vi "ge_GraphTblFGV.vi"(3 "ge_DAQManDefinitions":T1, 4 "Cal Ref":cluster{"EU RMS":dbl, "dB":bool}, 5 "ItemNames":string[][](array[string]), 6 "RMS Value":dbl, 7 "GrphTblCmnds":T4, 8 "error in":errorcluster, 9 "Legend LB":i32[](array[numeric]), 10 "Wfm In":waveform(dbl)[](array[waveform]), 11 "Init Info":T2) -> (0 "error out":errorcluster, 1 "Cell Contents":T3(array[cluster]), 2 "Wfm Out":waveform(dbl)[](array[waveform]))   [LabVIEW 2018]
uses:
  ge_GrphTblCmnds.ctl
  Classes/Measurements/Class Dynamic/Dynamic.lvclass
  C:/Users/Jeff Tipps/Documents/DAQMan/source/Classes/Measurements/Class Channel/Channel.lvclass
  Common/Controls/DAQMan Definitions.ctl
  Custom Ctrls/ge_FPCtrlRefLabel.ctl
  <vilib>/Utility/miscctls.llb/LVRowAndColumnTypeDef.ctl
  <vilib>/addons/_NISVFA/_Shared subVIs/Controls/svc_Channel Info.ctl
  <vilib>/addons/_NISVFA/_Shared subVIs/Controls/svc_Engineering Units Text Ring.ctl
  <vilib>/addons/_NISVFA/_Shared subVIs/Controls/svc_Weighting Filter Text Ring.ctl
  Custom Ctrls/ge_MeasType.ctl
  Common/Controls/HeaderNames.ctl
  <vilib>/addons/Sound and Vibration/svt_Calibration/SVL Scale Voltage to EU (1 Ch).vi
  <vilib>/addons/_NISVFA/_Shared subVIs/Common/svc_Set SV Channel Info.vi
  <vilib>/addons/_NISVFA/_Shared subVIs/Common/svc_Set SV Channel Info (variant).vi
  <vilib>/addons/_NISVFA/_Shared subVIs/Common/SVL Set dB Reference (variant).vi
  Classes/Measurements/Class Channel/Read Unit_EU.vi
  Classes/Measurements/Class Dynamic/Read dB Ref.vi
  <vilib>/addons/_NISVFA/_Shared subVIs/Common/svc_Engineering Units to Unit Label.vi
  <vilib>/addons/_NISVFA/_Shared subVIs/Common/svc_Compute Scale Factor to Convert V to EU.vi
  <vilib>/addons/_NISVFA/_Shared subVIs/Common/svc_Compute Scale Factor to Convert C to EU.vi
  <vilib>/addons/_NISVFA/_Shared subVIs/Common/svc_Set dB ref if Pascal.vi
  <vilib>/addons/_NISVFA/_Shared subVIs/Common/svc_Caller VI Returned in Error Source.vi
  Classes/Measurements/Class Dynamic/Read Cal Mag.vi
  Classes/Measurements/Class Dynamic/Read Cal Units.vi
  <vilib>/addons/Sound and Vibration/svt_Calibration/SoundVib_Calibration.lvlib
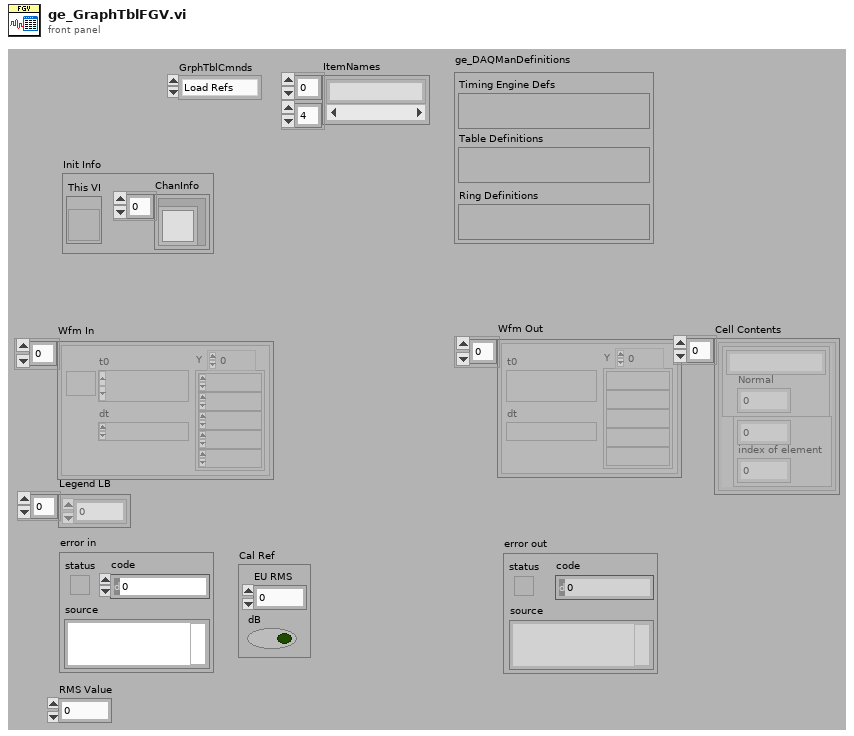
[diagram p1: front panel]
types:
  T1 = typedef "DAQMan Definitions.ctl" = cluster{"Timing Engine Defs":variant, "Table Definitions":variant, "Ring Definitions":variant}
  T2 = cluster{"This VI":refnum<vi>, "ChanInfo":refnum<class "Dynamic.lvclass">[]}
  T3 = cluster{cluster{string, "Normal":u32}, cluster{i32, "index of element":i32}}[]
  T4 = typedef "ge_GrphTblCmnds.ctl" = enum16{"Load Refs", "Init FP", "Active Plot", "CalRef", "AcceptCal", "Scale Wfm", "Update RMS", "Update Sens", "Get Sens", "Shutdown"}
  T5 = typedef "LVRowAndColumnTypeDef.ctl" = cluster{"Row":i32, "Column":i32}
  T6 = typedef "svc_Channel Info.ctl" = cluster{"sensor sensitivity":dbl, "engineering units":T7, "dB reference":dbl, "custom label":string, "weighting filter":T8, "pregain":dbl}
  T7 = typedef "svc_Engineering Units Text Ring.ctl" = u16
  T8 = typedef "svc_Weighting Filter Text Ring.ctl" = u16
  T9 = typedef "HeaderNames.ctl" = enum16{"Channel", "Device", "Spacer", "Description", "MB", "Range", "Terminal", "Coupling", "Thresh (V)", "Pulse/Rev", "Slope", "Min EU", "Min RPM", "mV/EU", "Iex", "Temp Units", "Type", "CJC Src", "CJC Val", "Ro", "Wire Cfg", "Strain Mode", "Vex", "Bridge Type", "GF", "Gauge Res", "Poisson", "Lead Res", "Init Strain", "GAF", "Scale", "Offset", "Unit (EU)", "dB?", "dB Ref", "Cal Mag", "Cal Units", "Max Temp", "Min Temp", "Max Strain", "Min Strain"}
  T10 = typedef "ge_MeasType.ctl" = enum16{"Voltage", "Frequency", "Tachometer", "Dynamic", "Thermocouple", "RTD", "Strain", "Current", "Resistance"}
  T11 = typedef "ge_FPCtrlRefLabel.ctl" = cluster{"Label Array":string[], "Ref Array":refnum<vi>[]}
  T12 = cluster{cluster{string, "Coerced":u32}, cluster{i32, "index of element":i32}}
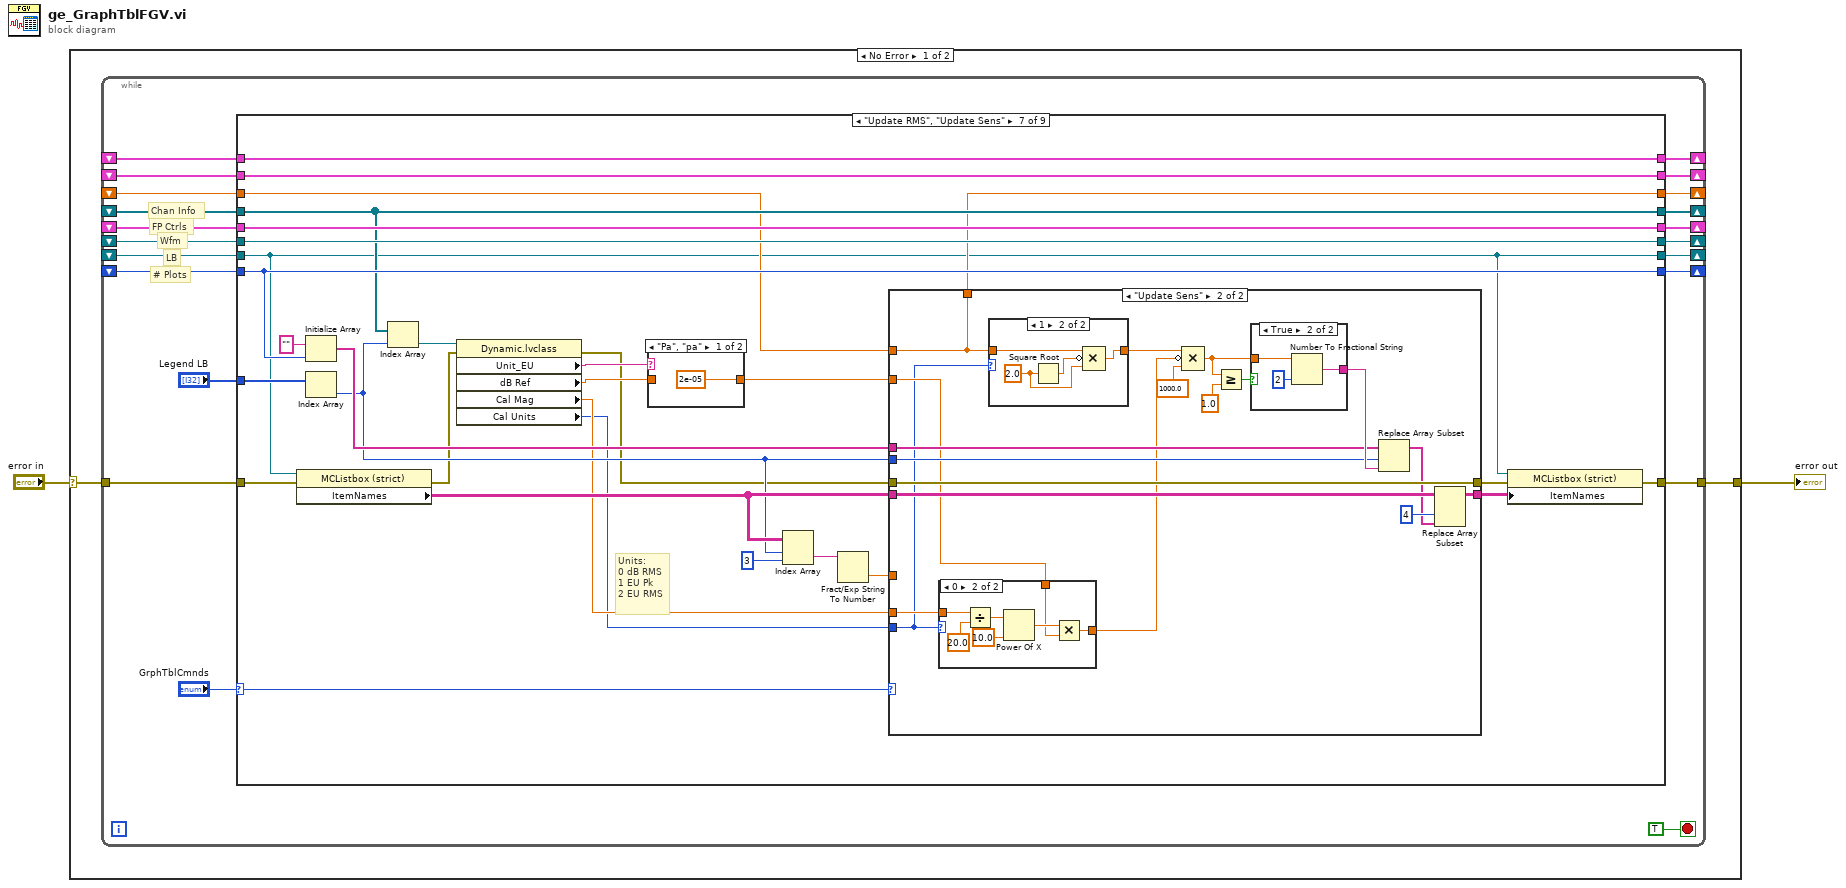
[diagram p0: block diagram]
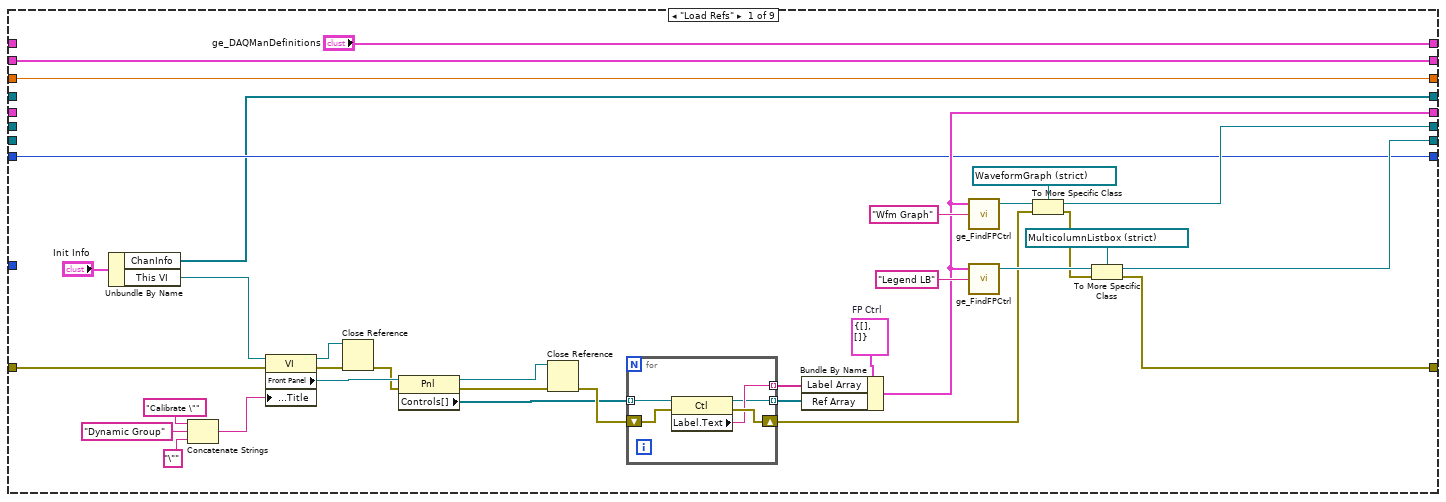
[diagram p2: hidden frame]
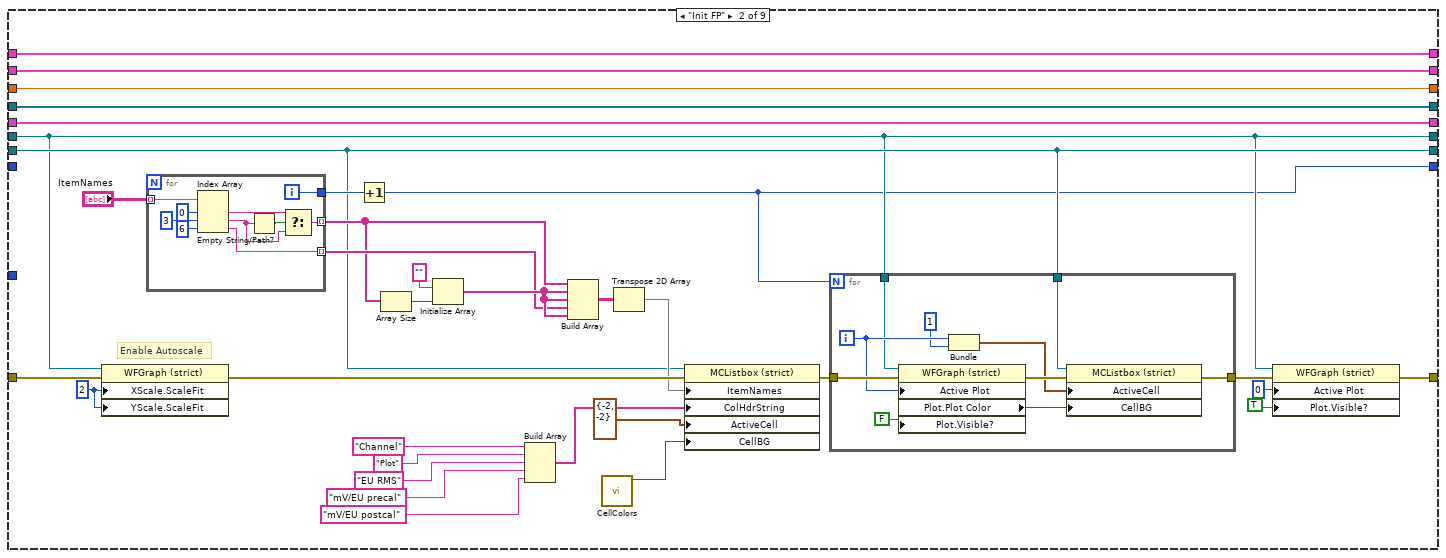
[diagram p3: hidden frame]
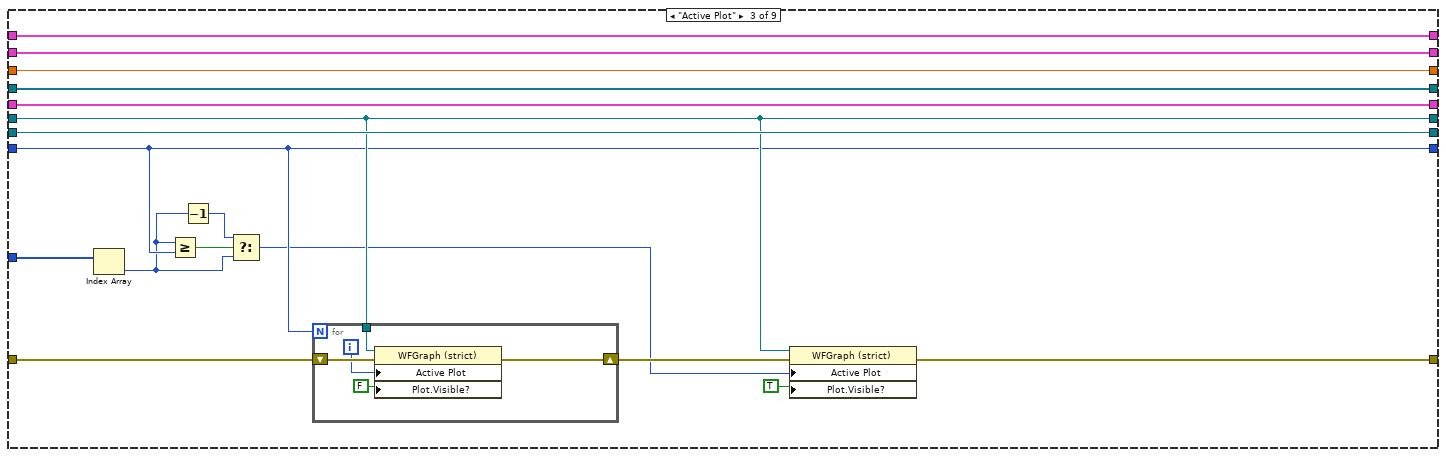
[diagram p4: hidden frame]
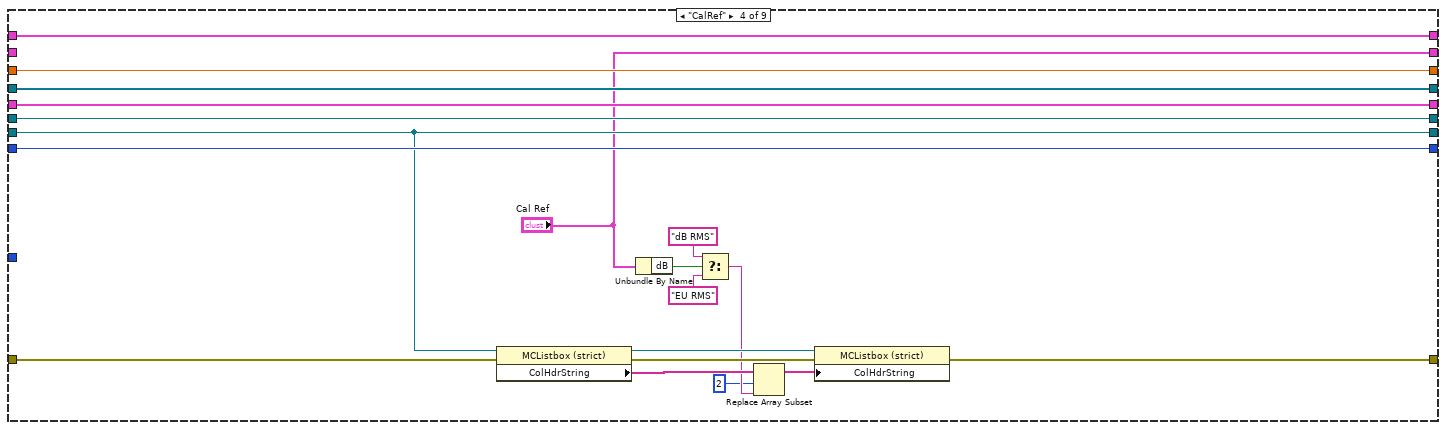
[diagram p5: hidden frame]
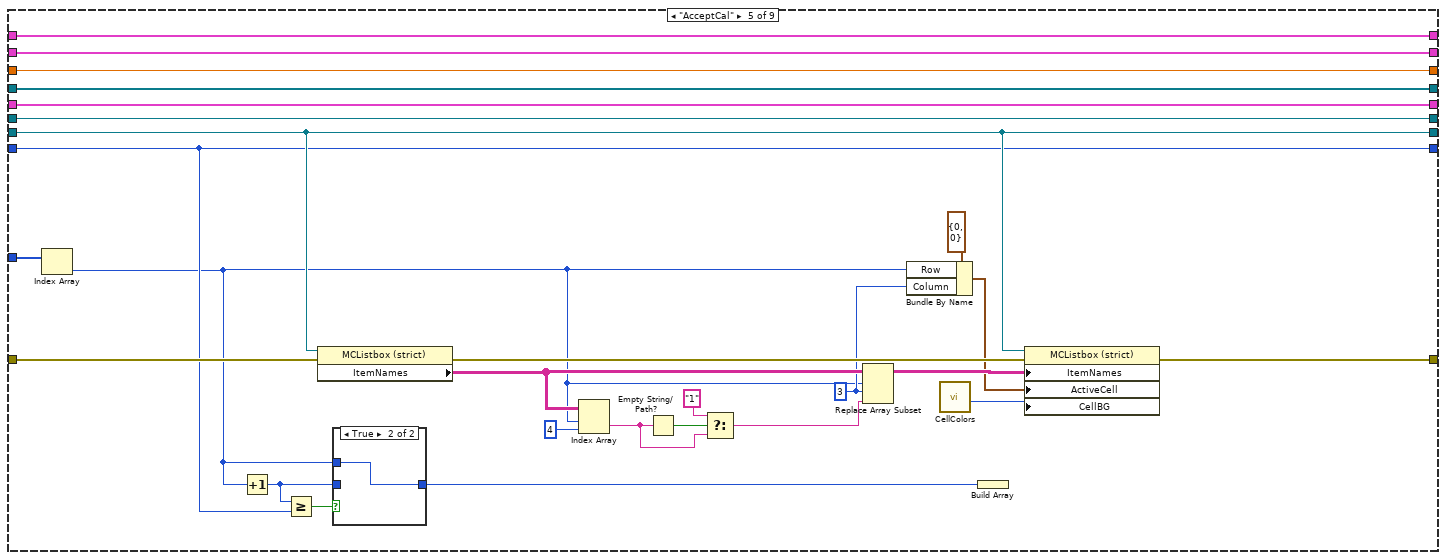
[diagram p6: hidden frame]
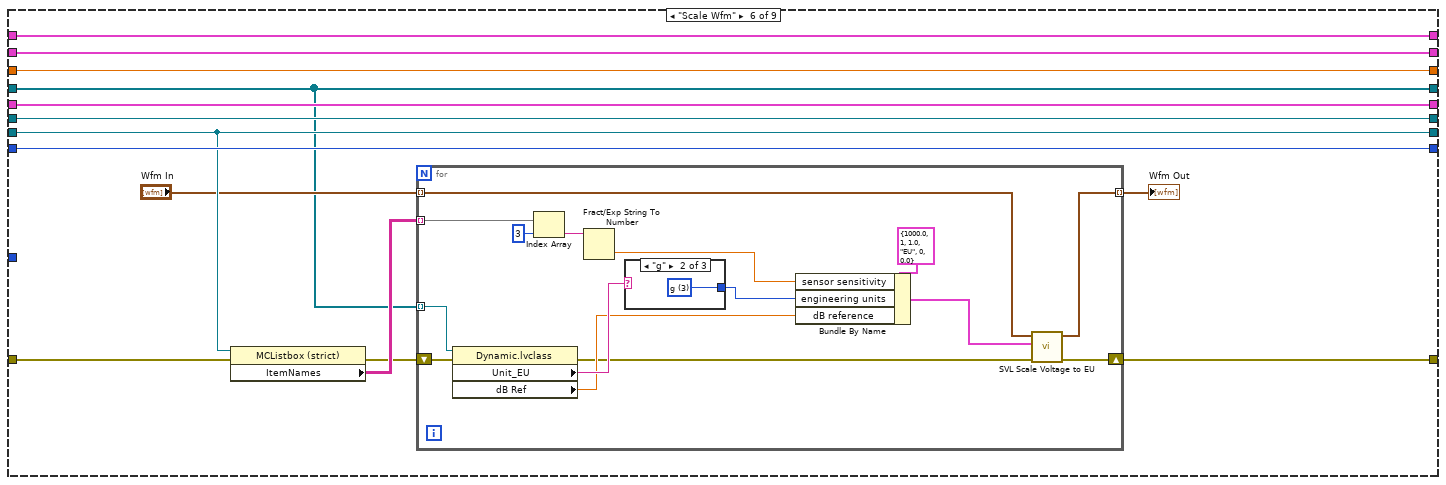
[diagram p8: hidden frame]
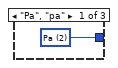
[diagram p9: hidden frame]
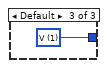
[diagram p10: hidden frame]
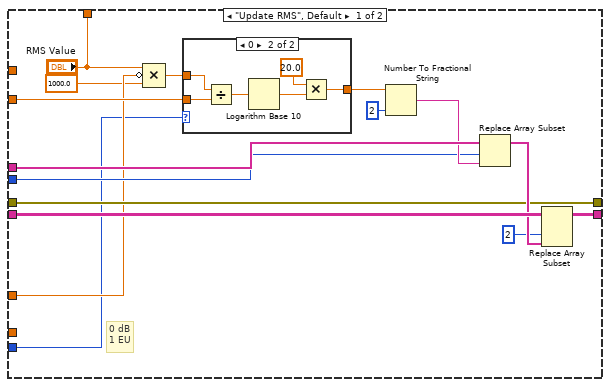
[diagram p11: hidden frame]
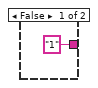
[diagram p15: hidden frame]
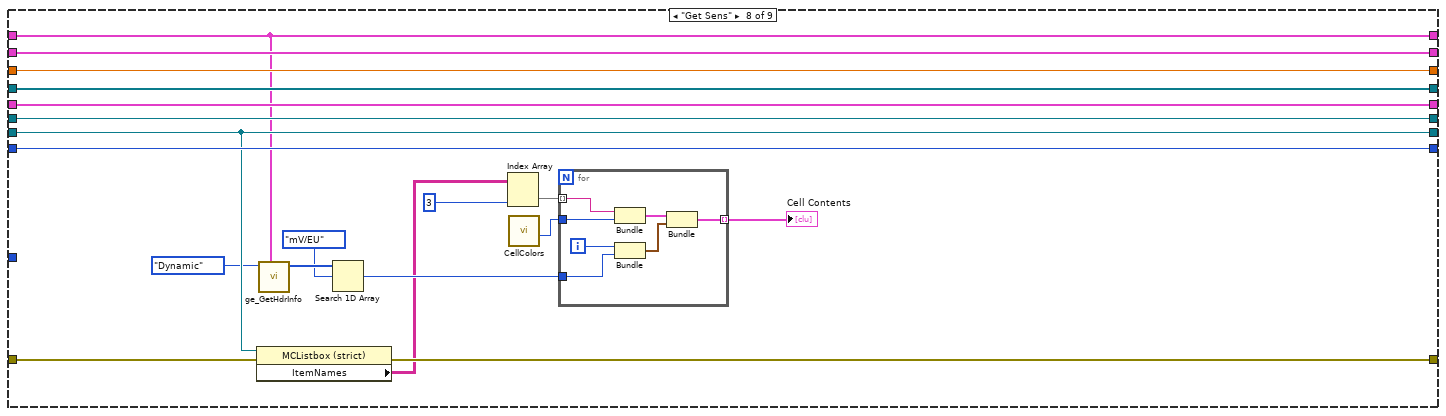
[diagram p17: hidden frame]
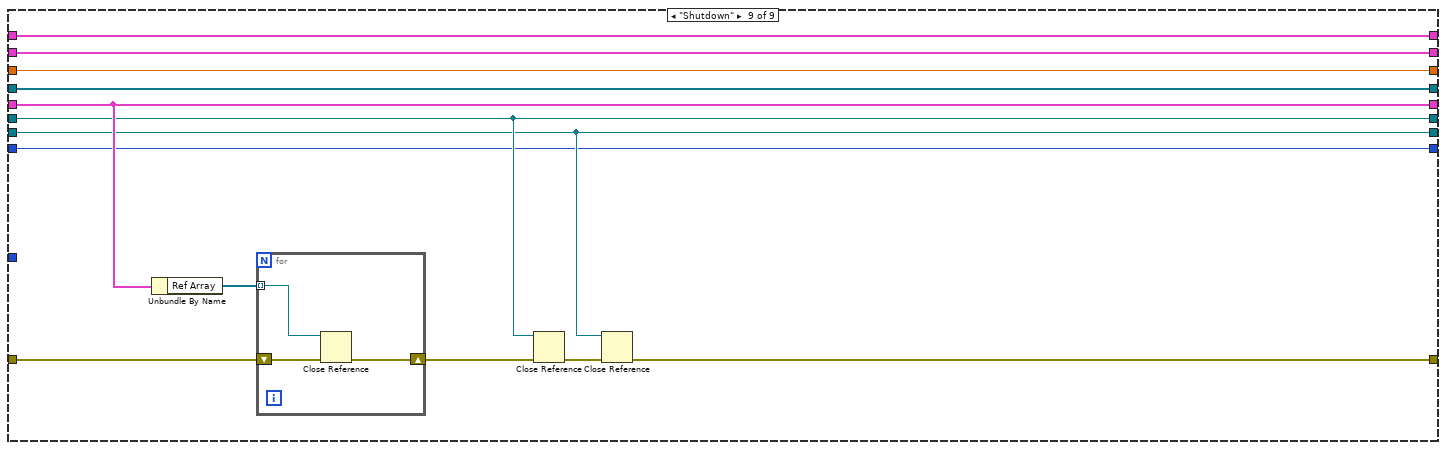
[diagram p18: hidden frame]
diagram:
  n1 = case shown="No Error" "error in" {
    selector: "error in" -> [w4 w353]
    tunnel: [w3 w353] -> w1
    frame No Error {
      n2 = while {
        tunnel: w4 -> [w25]
        tunnel: [w22] -> w3
        shift-right: [w21] -> _
        shift-left: _ -> [w19]
        shift-right: [w20] -> _
        shift-left: _ -> [w18]
        shift-right: [w17] -> _
        shift-left: _ -> [w16]
        shift-right: [w15] -> _
        shift-left: _ -> [w14]
        shift-right: [w12] -> _
        shift-left: _ -> [w11]
        shift-right: [w10] -> _
        shift-left: _ -> [w9]
        shift-right: [w8] -> _
        shift-left: _ -> [w7]
        shift-right: [w6] -> _
        shift-left: _ -> [w5]
        stop <- TRUE stop-if-true
        # "FP Ctrls"
        # "Chan Info"
        # "# Plots"
        # "Wfm"
        # "LB"
        n3 = case shown="\"Update RMS\", \"Update Sens\"" "GrphTblCmnds" {
          selector: "GrphTblCmnds" -> [_ _ _ _ _ _ w237 _ _]
          tunnel: w25 -> [w48 w97 w132 w154 w180 w199 w225 w324 w349]
          tunnel: [w38 w71 w135 w150 w179 w191 w243 w323 w344] -> w22
          tunnel: [w37 w72 w130 w158 w175 w201 w249 w328 w343] -> w21
          tunnel: [w35 w76 w133 w153 w178 w198 w236 w322 w342] -> w20
          tunnel: w19 -> [_ w72 w130 w158 w175 w201 w249 w328 w343]
          tunnel: w18 -> [_ w76 w133 w153 w178 w198 w236 w322 w342]
          tunnel: [w34 w98 w134 w159 w186 w202 w250 w329 w347] -> w17
          tunnel: w16 -> [_ w98 w134 w159 w186 w202 w250 w329 w347]
          tunnel: [w33 w70 w126 w157 w170 w200 w247 w327 w341] -> w15
          tunnel: w14 -> [w33 _ w126 w157 w170 w200 w247 w327 w341]
          tunnel: "Legend LB" -> [_ _ w127 _ w181 _ w246 _ _]
          tunnel: [w29 w69 w129 w156 w177 w190 w242 w326 w340] -> w12
          tunnel: w11 -> [_ w69 w129 w156 w177 w190 w242 w326 w340]
          tunnel: [w32 w68 w128 w155 w176 w195 w240 w325 w339] -> w10
          tunnel: w9 -> [w32 w68 w128 w155 w176 w195 w238 w325 w339]
          tunnel: [w28 w67 w120 "Cal Ref" w161 w194 w230 w316 w338] -> w8
          tunnel: w7 -> [w28 w67 w120 _ w161 w194 w230 w316 w338]
          tunnel: ["ge_DAQManDefinitions" w66 w119 w141 w160 w189 w229 w314 w337] -> w6
          tunnel: w5 -> [_ w66 w119 w141 w160 w189 w229 w314 w337]
          frame "Load Refs" {
            w49 = T11 {"Label Array"=[], "Ref Array"=[]}  # FP Ctrl
            n4 = Unbundle By Name("Init Info") -> ("ChanInfo"=w29:refnum<class "Dynamic.lvclass">[], "This VI"=w30:refnum<vi>)
            n5 = Concatenate Strings("Calibrate \"", "Dynamic Group" ("string"), "\"") -> (w52:string)
            n6 = property class="VI"(reference=w30, error in=w48, "Front Panel.Title"=w52) -> (reference out=w46:refnum<vi>, error out=w47:errorcluster, "Front Panel"=w56:refnum<vi>)
            n7 = Close Reference(reference=w46, error in (no error)=w47) -> (error out=w45:errorcluster)
            n8 = property class="Pnl"(reference=w56, error in=w45) -> (reference out=w60:refnum<vi>, error out=w58:errorcluster, "Controls[]"=w57:refnum<vi>[])
            n9 = Close Reference(reference=w60, error in (no error)=w58) -> (error out=w59:errorcluster)
            n10 = for {
              tunnel: w57 -> [w65] mode=indexing
              shift-right: [w63] -> w40
              shift-left: w59 -> [w64]
              tunnel: [w62] -> w51 mode=indexing
              tunnel: [w61] -> w50 mode=indexing
              n11 = property class="Ctl"(reference=w65, error in=w64) -> (reference out=w61:refnum<vi>, error out=w63:errorcluster, "Label.Text"=w62:string)
            }
            n12 = Bundle By Name(cluster=w49, "Label Array"=w51, "Ref Array"=w50) -> (w34:T11)
            n13 = call "ge_FindFPCtrl.vi"("Ctrl Name"="Wfm Graph", "FP Ctrl"=w34) -> ("Ctrl Ref"=w42:refnum<vi>)  [unwired: 3 in]
            n14 = call "ge_FindFPCtrl.vi"("Ctrl Name"="Legend LB", "FP Ctrl"=w34) -> ("Ctrl Ref"=w41:refnum<vi>)  [unwired: 3 in]
            n15 = To More Specific Class(target class=refnum<vi> refnum ("Wfm Graph"), reference=w42, error in=w40) -> (specific class reference=w37:refnum<vi>, error out=w39:errorcluster)
            n16 = To More Specific Class(target class=refnum<vi> refnum ("Legend LB"), reference=w41, error in=w39) -> (specific class reference=w35:refnum<vi>, error out=w38:errorcluster)
          }
          frame "Init FP" {
            w96 = u8 2 ("X Scale.Scale Fit")
            # "Enable Autoscale"
            n17 = property on="Property Node" class="WFGraph (strict)"(reference=w72, error in=w97, "XScale.ScaleFit"=w96, "YScale.ScaleFit"=w96) -> (error out=w95:errorcluster)  [unwired: 1 out]
            n18 = for {
              tunnel: "ItemNames" -> [w116] mode=indexing
              tunnel: [w117] -> w83 mode=indexing
              tunnel: [w110] -> w85 mode=indexing
              tunnel: [w109] -> w79
              i -> [w109]
              n19 = Index Array(array=w116, index #1=0 ("index"), index #2=3 ("index"), index #3=6 ("index")) -> (element #1=w114:string, element #2=w113:string, element #3=w110:string)
              n20 = Empty String/Path?(string/path=w113) -> (empty?=w118:bool)
              n21 = Select(t=w114, s=w118, f=w113) -> (s? t:f=w117:string)
            }
            n22 = Increment(x=w79) -> (x+1=w70:i32)
            n23 = Array Size(array=w83) -> (size(s)=w82:i32)
            n24 = Initialize Array("", w82) -> (w86:string[])
            n25 = Build Array("Channel", "Plot", "EU RMS", "mV/EU precal" ("element"), "mV/EU postcal" ("element")) -> (w89:string[])
            n26 = Build Array(w83, w86, w86, w85, w86) -> (w84:string[][])
            n27 = call "CellColors.vi"() -> ("Normal"=w87:u32)  [unwired: 8 in, 3 out]
            n28 = Transpose 2D Array(2D array=w84) -> (transposed array=w77:string[][])
            n29 = property on="Property Node" class="MCListbox (strict)"(reference=w76, error in=w95, "ItemNames"=w77, "ColHdrString"=w89, "ActiveCell"=T5 {"Row"=-2, "Column"=-2} ("Active Cell:Active Cell"), "CellBG"=w87) -> (error out=w78:errorcluster)  [unwired: 1 out]
            n30 = for {
              N: w70 -> [_]
              tunnel: [w108] -> w73
              tunnel: w78 -> [w106]
              tunnel: w72 -> [w100]
              tunnel: w76 -> [w99]
              i -> [w104]
              n31 = property on="Property Node" class="WFGraph (strict)"(reference=w100, error in=w106, "Active Plot"=w104, "Plot.Visible?"=FALSE ("Plot.Visible")) -> (error out=w107:errorcluster, "Plot.Plot Color"=w105:u32)  [unwired: 1 out]
              n32 = Bundle(w104, 1) -> (w102:cluster{i32, i32})  [unwired: 1 in]
              n33 = property on="Property Node" class="MCListbox (strict)"(reference=w99, error in=w107, "ActiveCell"=w102, "CellBG"=w105) -> (error out=w108:errorcluster)  [unwired: 1 out]
            }
            n34 = property on="Property Node" class="WFGraph (strict)"(reference=w72, error in=w73, "Active Plot"=u32 0, "Plot.Visible?"=TRUE ("Plot.Visible")) -> (error out=w71:errorcluster)  [unwired: 1 out]
          }
          frame "Active Plot" {
            n35 = Index Array(array=w127) -> (element=w124:i32)  [unwired: 1 in]
            n36 = Greater Or Equal?(x=w124, y=w126) -> (x >= y?=w125:bool)
            n37 = Decrement(x=w124) -> (x-1=w123:i32)
            n38 = Select(t=w123, s=w125, f=w124) -> (s? t:f=w122:i32)
            n39 = for {
              N: w126 -> [_]
              shift-right: [w139] -> w131
              shift-left: w132 -> [w140]
              tunnel: w130 -> [w136]
              i -> [w137]
              n40 = property on="Property Node" class="WFGraph (strict)"(reference=w136, error in=w140, "Active Plot"=w137, "Plot.Visible?"=FALSE ("Plot.Visible")) -> (error out=w139:errorcluster)  [unwired: 1 out]
            }
            n41 = property on="Property Node" class="WFGraph (strict)"(reference=w130, error in=w131, "Active Plot"=w122, "Plot.Visible?"=TRUE ("Plot.Visible")) -> (error out=w135:errorcluster)  [unwired: 1 out]
          }
          frame "CalRef" {
            n42 = property on="Property Node" class="MCListbox (strict)"(reference=w153, error in=w154) -> (reference out=w147:refnum<vi>, error out=w151:errorcluster, "ColHdrString"=w148:string[])
            n43 = Unbundle By Name("Cal Ref") -> ("dB"=w149:bool)
            n44 = Select(t="dB RMS", s=w149, f="EU RMS") -> (s? t:f=w146:string)
            n45 = Replace Array Subset(array=w148, new element=w146, index=2) -> (w142:string[])
            n46 = property on="Property Node" class="MCListbox (strict)"(reference=w147, error in=w151, "ColHdrString"=w142) -> (error out=w150:errorcluster)  [unwired: 1 out]
          }
          frame "AcceptCal" {
            w173 = 3 ("disabled index (col)")
            n47 = Index Array(array=w181) -> (element=w168:i32)  [unwired: 1 in]
            n48 = Increment(x=w168) -> (x+1=w166:i32)
            n49 = Greater Or Equal?(x=w166, y=w170) -> (x >= y?=w169:bool)
            n50 = property on="Property Node" class="MCListbox (strict)"(reference=w178, error in=w180) -> (error out=w184:errorcluster, "ItemNames"=w183:string[][])  [unwired: 1 out]
            n51 = case shown="True" w169 {
              tunnel: w168 -> [_ w188]
              tunnel: [w187 w188] -> w167
              tunnel: w166 -> [w187 _]
              frame False {
              }
              frame True {
              }
            }
            n52 = Index Array(array=w183, index (row)=w168, index (col)=4 ("disabled index (col)")) -> (element=w164:string)
            n53 = Empty String/Path?(string/path=w164) -> (empty?=w165:bool)
            n54 = Select(t="1", s=w165, f=w164) -> (s? t:f=w162:string)
            n55 = Replace Array Subset(array=w183, new element=w162, index (row)=w168, index (col)=w173) -> (w185:string[][])
            n56 = Bundle By Name(cluster=T5 {"Row"=0, "Column"=0} ("Active Cell:Active Cell"), "Row"=w168, "Column"=w173) -> (w172:T5)
            n57 = call "CellColors.vi"() -> ("Coerced"=w171:u32)  [unwired: 8 in, 3 out]
            n58 = Build Array(w167) -> ()  [unwired: 1 out]
            n59 = property on="Property Node" class="MCListbox (strict)"(reference=w178, error in=w184, "ItemNames"=w185, "ActiveCell"=w172, "CellBG"=w171) -> (error out=w179:errorcluster)  [unwired: 1 out]
          }
          frame "Scale Wfm" {
            n60 = property on="Property Node" class="MCListbox (strict)"(reference=w198, error in=w199) -> (error out=w192:errorcluster, "ItemNames"=w197:string[][])  [unwired: 1 out]
            n61 = for {
              tunnel: w197 -> [w217] mode=indexing
              tunnel: "Wfm In" -> [w212] mode=indexing
              tunnel: [w213] -> w193 mode=indexing
              shift-right: [w214] -> w191
              shift-left: w192 -> [w207]
              tunnel: w190 -> [w206] mode=indexing
              n62 = property class="Dynamic.lvclass"(reference=w206, error in=w207) -> (error out=w203:errorcluster, "Unit_EU"=w205:string, "dB Ref"=w204:dbl)  [unwired: 1 out]
              n63 = Index Array(array=w217, index=3) -> (element=w215:string)
              n64 = Fract/Exp String To Number(string=w215) -> (number=w210:dbl)  [unwired: 3 in, 1 out]
              n65 = case shown="\"g\"" w205 {
                tunnel: [w218 w219 w220] -> w208
                frame "Pa", "pa" {
                  w218 = T7 2 items=["custom..."=0, "V"=1, "A"=21, "Pa"=2, "N"=20, "g"=3, "m/s^2"=4, "m/s"=5, "m"=6, "mm/s"=12, "mm"=13, "micron/s"=14, "micron"=15, "in/s^2"=7, "in/s"=8, "in"=9, "mil/s"=10, "mil"=11, "rad/s^2"=16, "rad/s"=17, "rad"=18, "deg/s^2"=26, "deg/s"=27, "deg"=28, "RPM"=22, "cycle/s^2"=23, "Hz"=24, "cycle"=25, "strain"=19] ("engineering units")
                }
                frame "g" {
                  w219 = T7 3 items=["custom..."=0, "V"=1, "A"=21, "Pa"=2, "N"=20, "g"=3, "m/s^2"=4, "m/s"=5, "m"=6, "mm/s"=12, "mm"=13, "micron/s"=14, "micron"=15, "in/s^2"=7, "in/s"=8, "in"=9, "mil/s"=10, "mil"=11, "rad/s^2"=16, "rad/s"=17, "rad"=18, "deg/s^2"=26, "deg/s"=27, "deg"=28, "RPM"=22, "cycle/s^2"=23, "Hz"=24, "cycle"=25, "strain"=19] ("engineering units")
                }
                frame Default {
                  w220 = T7 1 items=["custom..."=0, "V"=1, "A"=21, "Pa"=2, "N"=20, "g"=3, "m/s^2"=4, "m/s"=5, "m"=6, "mm/s"=12, "mm"=13, "micron/s"=14, "micron"=15, "in/s^2"=7, "in/s"=8, "in"=9, "mil/s"=10, "mil"=11, "rad/s^2"=16, "rad/s"=17, "rad"=18, "deg/s^2"=26, "deg/s"=27, "deg"=28, "RPM"=22, "cycle/s^2"=23, "Hz"=24, "cycle"=25, "strain"=19] ("engineering units")
                }
              }
              n66 = Bundle By Name(cluster=T6 {"sensor sensitivity"=1000.0, "engineering units"=1, "dB reference"=1.0, "custom label"="EU", "weighting filter"=0, "pregain"=0.0} ("channel info"), "sensor sensitivity"=w210, "engineering units"=w208, "dB reference"=w204) -> (w209:T6)
              n67 = call-poly <vilib>:"SVL Scale Voltage to EU.vi"("error in (no error)"=w203, "channel info"=w209, "signal [V]"=w212) -> ("error out"=w214:errorcluster, "scaled signal [EU]"=w213:waveform(dbl))  [unwired: 6 in, 1 out]
            }
            "Wfm Out" <- w193
          }
          frame "Update RMS", "Update Sens" {
            # "Units:\n0 dB RMS\n1 EU Pk\n2 EU RMS"
            n68 = property on="Property Node" class="MCListbox (strict)"(reference=w236, error in=w225) -> (error out=w222:errorcluster, "ItemNames"=w233:string[][])  [unwired: 1 out]
            n69 = Initialize Array("", w247) -> (w245:string[])
            n70 = Index Array(array=w246) -> (element=w232:i32)  [unwired: 1 in]
            n71 = Index Array(array=w242, index=w232) -> (element=w228:refnum<class "Dynamic.lvclass">)
            n72 = property class="Dynamic.lvclass"(reference=w228, error in=w222) -> (error out=w221:errorcluster, "Unit_EU"=w227:string, "dB Ref"=w226:dbl, "Cal Mag"=w224:dbl, "Cal Units"=w223:u16)  [unwired: 1 out]
            n73 = case shown="\"Pa\", \"pa\"" w227 {
              tunnel: w226 -> [_ w310]
              tunnel: [2e-05 ("dB Ref") w310] -> w241
              frame "Pa", "pa" {
              }
              frame Default {
              }
            }
            n74 = Index Array(array=w233, index (row)=w232, index (col)=3 ("disabled index (col)")) -> (element=w234:string)
            n75 = Fract/Exp String To Number(string=w234) -> (number=w231:dbl)  [unwired: 3 in, 1 out]
            n76 = case shown="\"Update Sens\"" w237 {
              tunnel: w245 -> [w265 w282]
              tunnel: w233 -> [w264 w290]
              tunnel: [w262 w289] -> w244
              tunnel: w241 -> [w259 w277]
              tunnel: w232 -> [w257 w281]
              tunnel: ["RMS Value" w276] -> w240
              tunnel: [w256 w291] -> w239
              tunnel: w221 -> [w256 w291]
              tunnel: w238 -> [_ w276]
              tunnel: w231 -> [w254 _]
              tunnel: w224 -> [_ w278]
              tunnel: w223 -> [w251 w274]
              frame "Update RMS", Default {
                # "0 dB\n1 EU"
                n77 = Compound Arithmetic op=MULTIPLY("RMS Value", invert w254, 1000.0 ("value")) -> (w253:dbl)
                n78 = case shown="0" w251 {
                  tunnel: w259 -> [_ w273]
                  tunnel: [w267 w269] -> w258
                  tunnel: w253 -> [w267 w268]
                  frame 1, Default {
                  }
                  frame 0 {
                    n79 = Divide(x=w268, y=w273) -> (x/y=w272:dbl)
                    n80 = Logarithm Base 10(1:w272) -> (0:w271:dbl)
                    n81 = Multiply(x=20.0, y=w271) -> (x*y=w269:dbl)
                  }
                }
                n82 = Number To Fractional String(number=w258, precision (6)=i16 2) -> (F-format string=w260:string)  [unwired: 2 in]
                n83 = Replace Array Subset(array=w265, new element=w260, index=w257) -> (w263:string[])
                n84 = Replace Array Subset(array=w264, new element=w263, index (col)=2 ("disabled index (col)")) -> (w262:string[][])  [unwired: 1 in]
              }
              frame "Update Sens" {
                n85 = case shown="0" w274 {
                  tunnel: w277 -> [_ w300]
                  tunnel: [w297 w299] -> w279
                  tunnel: w278 -> [w297 w298]
                  frame Default {
                  }
                  frame 0 {
                    n86 = Divide(x=w298, y=20.0) -> (x/y=w302:dbl)
                    n87 = Power Of X(1:10.0 ("x"), 2:w302) -> (0:w303:dbl)
                    n88 = Multiply(x=w303, y=w300) -> (x*y=w299:dbl)
                  }
                }
                n89 = case shown="1" w274 {
                  tunnel: w276 -> [w292 w296]
                  tunnel: [w292 w293] -> w275
                  frame Default {
                  }
                  frame 1 {
                    w294 = 2.0 ("x")
                    n90 = Square Root(x=w294) -> (sqrt(x)=w295:dbl)
                    n91 = Compound Arithmetic op=MULTIPLY(w296, invert w295, w294) -> (w293:dbl)
                  }
                }
                n92 = Compound Arithmetic op=MULTIPLY(w275, invert w279, 1000.0 ("value")) -> (w287:dbl)
                n93 = Greater Or Equal?(x=w287, y=1.0) -> (x >= y?=w285:bool)
                n94 = case shown="True" w285 {
                  tunnel: ["1" w307] -> w283
                  tunnel: w287 -> [_ w306]
                  frame False {
                  }
                  frame True {
                    n95 = Number To Fractional String(number=w306, precision (6)=i16 2) -> (F-format string=w307:string)  [unwired: 2 in]
                  }
                }
                n96 = Replace Array Subset(array=w282, new element=w283, index=w281) -> (w280:string[])
                n97 = Replace Array Subset(array=w290, new element=w280, index (col)=4 ("disabled index (col)")) -> (w289:string[][])  [unwired: 1 in]
              }
            }
            n98 = property on="Property Node" class="MCListbox (strict)"(reference=w236, error in=w239, "ItemNames"=w244) -> (error out=w243:errorcluster)  [unwired: 1 out]
          }
          frame "Get Sens" {
            n99 = property on="Property Node" class="MCListbox (strict)"(reference=w322, error in=w324) -> (error out=w323:errorcluster, "ItemNames"=w313:string[][])  [unwired: 1 out]
            n100 = call "ge_GetHdrInfo.vi"("ge_DAQManDefinitions"=w314, "MeasType"=ge_MeasType."Dynamic") -> ("Hdr Name"=w319:T9[])  [unwired: 7 in, 2 out]
            n101 = Search 1D Array(1D array=w319, element=HeaderNames."mV/EU" ("ge_HdrNames")) -> (index of element=w318:i32)  [unwired: 1 in]
            n102 = Index Array(array=w313, index (col)=3 ("disabled index (col)")) -> (element=w321:string[])  [unwired: 1 in]
            n103 = call "CellColors.vi"() -> ("Coerced"=w315:u32)  [unwired: 8 in, 3 out]
            n104 = for {
              tunnel: w321 -> [w336] mode=indexing
              tunnel: w315 -> [w335]
              tunnel: w318 -> [w333]
              tunnel: [w330] -> w317 mode=indexing
              i -> [w334]
              n105 = Bundle(w336, "Coerced"=w335) -> (w332:cluster{string, "Coerced":u32})  [unwired: 1 in]
              n106 = Bundle(w334, "index of element"=w333) -> (w331:cluster{i32, "index of element":i32})  [unwired: 1 in]
              n107 = Bundle(w332, w331) -> (w330:T12)  [unwired: 1 in]
            }
            "Cell Contents" <- w317
          }
          frame "Shutdown" {
            n108 = Unbundle By Name(w347) -> ("Ref Array"=w348:refnum<vi>[])
            n109 = for {
              tunnel: w348 -> [w350] mode=indexing
              shift-right: [w351] -> w346
              shift-left: w349 -> [w352]
              n110 = Close Reference(reference=w350, error in (no error)=w352) -> (error out=w351:errorcluster)
            }
            n111 = Close Reference(reference=w343, error in (no error)=w346) -> (error out=w345:errorcluster)
            n112 = Close Reference(reference=w342, error in (no error)=w345) -> (error out=w344:errorcluster)
          }
        }
      }
    }
    frame Error {
    }
  }
  "error out" <- w1
